vi "Build Methods.vi"(8 "error in (no error)":errorcluster, 9 "ProgressBarCluster":T1, 10 "Wiring Spec":T2, 11 "CS++Actor in":refnum<class "CS++Actor.lvclass">) -> (0 "error out":errorcluster, 3 "CS++Actor out":refnum<class "CS++Actor.lvclass">)   [LabVIEW 2014, in "CS++Actor.lvlib" / "CS++Actor.lvclass"]
doc: "Creates the methods for the new message."
uses:
  CS++Actor.lvclass
  CS++Actor.lvclass/CS++Actor.ctl
  CSPP_MessageMaker_Utilities/CS++MessagemakerUtilities.lvlib
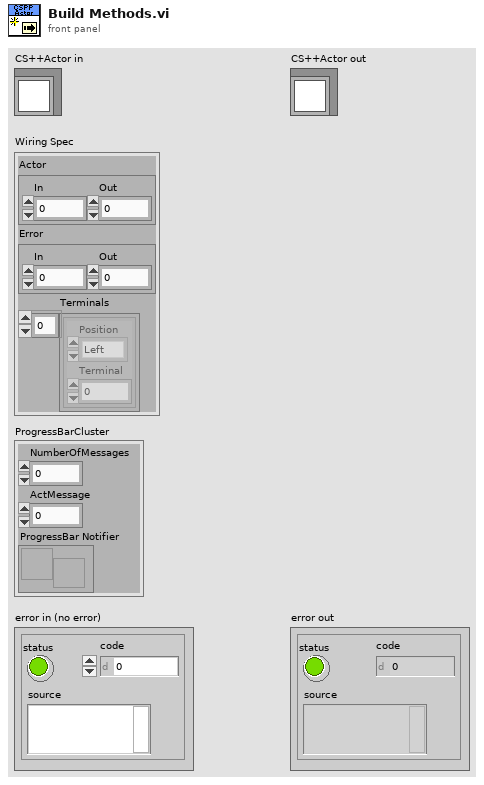
[diagram p1: front panel]
types:
  T1 = cluster{"NumberOfMessages":u16, "ActMessage":u16, "ProgressBar Notifier":refnum<notifier>}
  T2 = cluster{"Actor":cluster{"In":i32, "Out":i32}, "Error":cluster{"In":i32, "Out":i32}, "Terminals":cluster{"Position":enum16{"Left", "Top", "Bottom", "Right"}, "Terminal":i32}[]}
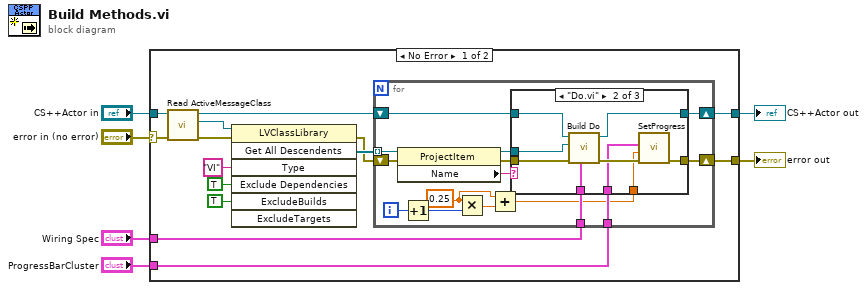
[diagram p0: block diagram]
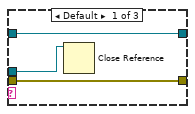
[diagram p2: hidden frame]
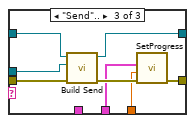
[diagram p3: hidden frame]
diagram:
  n1 = case shown="No Error" "error in (no error)" {
    selector: "error in (no error)" -> [w10 w57]
    tunnel: [w15 w57] -> w5
    tunnel: [w13 w56] -> w3
    tunnel: "CS++Actor in" -> [w11 w56]
    tunnel: "Wiring Spec" -> [w14 _]
    tunnel: "ProgressBarCluster" -> [w7 _]
    frame No Error {
      n2 = call "Read ActiveMessageClass.vi"("error in (no error)"=w10, "CS++Actor in"=w11) -> ("error out"=w8:errorcluster, "ActiveMessageClass"=w12:refnum<vi>, "CS++Actor out"=w9:refnum<class "CS++Actor.lvclass">)  [unwired: 7 in]
      n3 = invoke class="LVClassLibrary" method="Get All Descendents"(reference=w12, error in=w8, "Type"="VI", "Exclude Dependencies"=TRUE ("ExcludeDependencies"), "ExcludeBuilds"=TRUE) -> (error out=w16:errorcluster, "All Descendents"=w17:refnum<vi>[])  [unwired: 2 in, 5 out]
      n4 = for {
        tunnel: w17 -> [w35] mode=indexing
        shift-right: [w32] -> w15
        shift-left: w16 -> [w34]
        tunnel: w14 -> [w29]
        shift-right: [w27] -> w13
        shift-left: w9 -> [w28]
        tunnel: w7 -> [w26]
        i -> [w25]
        w22 = 0.25 ("SubStep")
        n5 = property class="ProjectItem"(reference=w35, error in=w34) -> (reference out=w30:refnum<vi>, error out=w31:errorcluster, "Name"=w33:string)
        n6 = Increment(x=w25) -> (x+1=w24:i32)
        n7 = Multiply(x=w22, y=w24) -> (x*y=w23:dbl)
        n8 = Add(x=w22, y=w23) -> (x+y=w21:dbl)
        n9 = case shown="\"Do.vi\"" w33 {
          tunnel: [w38 w41 w50] -> w32
          tunnel: w31 -> [w38 w47 w55]
          tunnel: w30 -> [w37 w45 w52]
          tunnel: w29 -> [_ w46 _]
          tunnel: w28 -> [w36 w44 w54]
          tunnel: [w36 w43 w53] -> w27
          tunnel: w26 -> [_ w40 w49]
          tunnel: w21 -> [_ w39 w48]
          frame Default {
            n10 = Close Reference(reference=w37) -> ()  [unwired: 1 in, 1 out]
          }
          frame "Do.vi" {
            n11 = call "Build Do.vi"("Wiring Spec"=w46, "error in (no error)"=w47, "Do VI"=w45, "CS++Actor in"=w44) -> ("error out"=w42:errorcluster, "CS++Actor out"=w43:refnum<class "CS++Actor.lvclass">)  [unwired: 6 in]
            n12 = call "SetProgress.vi"("error in (no error)"=w42, "SubStep"=w39, "ProgressBarCluster"=w40) -> ("error out"=w41:errorcluster)  [unwired: 8 in]
          }
          frame "Send".. {
            n13 = call "Build Send.vi"("error in (no error)"=w55, "Send VI"=w52, "CS++Actor in"=w54) -> ("error out"=w51:errorcluster, "CS++Actor out"=w53:refnum<class "CS++Actor.lvclass">)  [unwired: 7 in]
            n14 = call "SetProgress.vi"("error in (no error)"=w51, "SubStep"=w48, "ProgressBarCluster"=w49) -> ("error out"=w50:errorcluster)  [unwired: 8 in]
          }
        }
      }
    }
    frame Error {
    }
  }
  "error out" <- w5
  "CS++Actor out" <- w3
